vi "PS90_GetReadError.vi"(3 "error in (no error)":errorcluster, 4 "Control unit ID":i32=1 min=1 max=10, 5 "DLOwis.lvclass":refnum<class "DLOwis.lvclass">) -> (0 "error IO":errorcluster, 1 "Read error":i32, 2 "DLOwis.lvclass":refnum<class "DLOwis.lvclass">)   [LabVIEW 2018]
doc: "PS90_GetReadError.vi, created: 10.10.2006 alex; last change: 22.07.2016 alex;\n\n<B>FUNCTION:</B> \n\nRead error code of the last read function (PS90_Get...).\n----------------------------------------------------------------------------------------\n<B>INPUT:</B>\n[I32] <B>Control unit ID:</B> control unit index. (Default=1, Range=1...10) \n----------------------------------------------------------------------------------------\n<B>OUTPUT:</B>\n[I32] <B>Read error:</B> error code of the last read function.\n 0 - function was successful (no error),\n-1 - function error,\n-2 - communication error,\n-3 - syntax error,\n-4 - axis in wrong state.\n----------------------------------------------------------------------------------------\n<B>SUB-VIs:</B>\n----------------------------------------------------------------------------------------\n<B>EXT-Calls:</B>\nps90.dll (V2.00)\n----------------------------------------------------------------------------------------"
uses:
  DLOwis.lvclass
  C:/Dev/TRANCON/Classes/Delay Line/DelayLine.lvclass
  DelayLine.lvclass/DelayLine.ctl
  DelayLine.lvclass
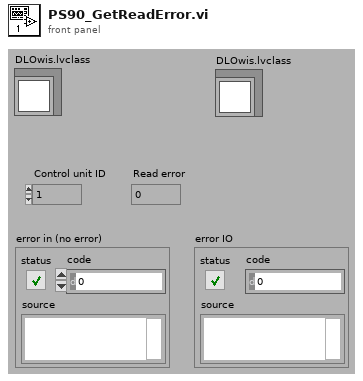
[diagram p1: front panel]
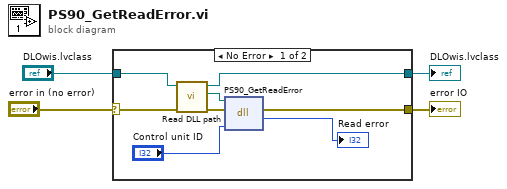
[diagram p0: block diagram]
diagram:
  n1 = case shown="No Error" "error in (no error)" {
    selector: "error in (no error)" -> [w7 w13]
    tunnel: [w8 w14] -> w3
    tunnel: "DLOwis.lvclass" -> [w9 w14]
    tunnel: [w10 w13] -> w1
    frame No Error {
      n2 = call "Read DLL path.vi"("error in (no error)"=w7, "DelayLine in"=w9) -> ("error out"=w6:errorcluster, "DLL path"=w5:path, "DelayLine out"=w8:refnum<class "DLOwis.lvclass">)  [unwired: 7 in]
      n3 = dll-call lib="C:/Dev/TRANCON/DLL/ps90.dll" fn="PS90_GetReadError"(path in=w5, error in=w6, "Index"="Control unit ID") -> (error out=w10:errorcluster, "Rückgabetyp"=→"Read error":i32)  [unwired: 2 in, 1 out]
    }
    frame Error {
    }
  }
  "DLOwis.lvclass" <- w3
  "error IO" <- w1
